vi "Get Container Metadata.vi"(8 "error in (no error)":errorcluster, 10 "Container":string, 11 "Azure Session in":refnum<class "Session.lvclass">) -> (0 "error out":errorcluster, 2 "Metadata":T1[](array[typedef]), 3 "Azure Session out":refnum<class "Session.lvclass">)   [LabVIEW 2015, in "NI_Azure_Blob.lvlib"]
doc: "Returns only user-defined metadata of a container."
uses:
  NI_Azure_Blob.lvlib
  Core/Session/Session.lvclass
  Core/Name Value Pair.ctl
  Core/Session/Session.lvclass/Session.ctl
  Core/Session/Write Request Parameters.vi
  Core/Session/Write HTTP Verb.vi
  Core/Session/Write URL Suffix.vi
  Core/NI_Azure_Core.lvlib
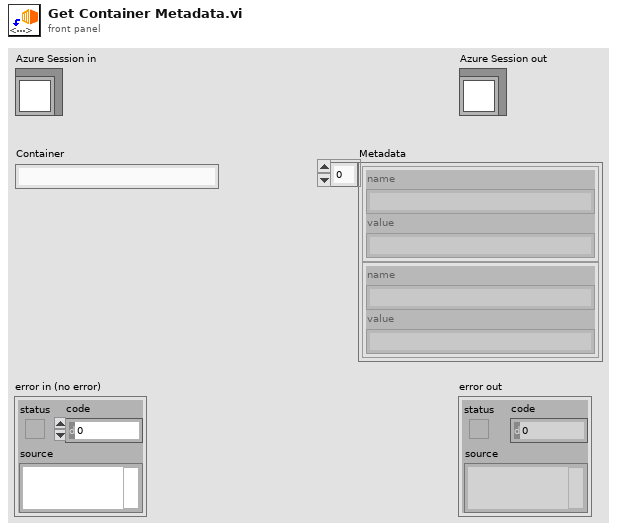
[diagram p1: front panel]
types:
  T1 = typedef "NI_Azure_Core.lvlib/Name Value Pair.ctl" = cluster{"name":string, "value":string}
  T2 = typedef "NI_Azure_Core.lvlib/Response.ctl" = cluster{"Headers":string, "Body":string}
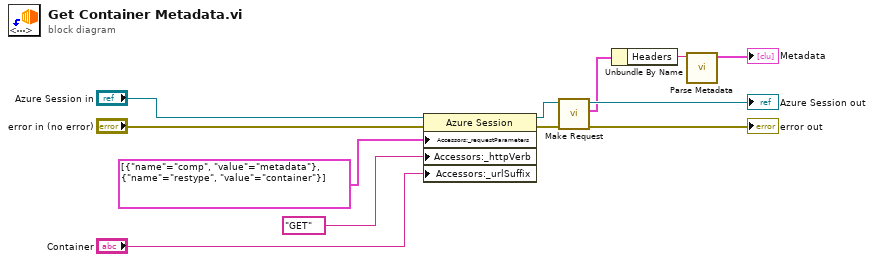
[diagram p0: block diagram]
diagram:
  n1 = property class="Azure Session"(reference="Azure Session in", error in="error in (no error)", "Accessors:_requestParameters"=T1[] [{"name"="comp", "value"="metadata"}, {"name"="restype", "value"="container"}] ("request parameters"), "Accessors:_httpVerb"="GET" ("HTTP-Verb"), "Accessors:_urlSuffix"="Container") -> (reference out=w4:refnum<class "Session.lvclass">, error out=w6:errorcluster)
  n2 = call "Make Request.vi"("error in (no error)"=w6, "Session in"=w4) -> ("error out"=→"error out":errorcluster, "Response"=w7:T2, "Session out"=→"Azure Session out":refnum<class "Session.lvclass">)  [unwired: 7 in]
  n3 = Unbundle By Name(w7) -> ("Headers"=w8:string)
  n4 = call "Parse Metadata.vi"("String"=w8) -> ("Metadata"=→"Metadata":T1[])  [unwired: 10 in]
